vi "Enqeue message camera.vi"(8 "error in (no error)":errorcluster, 11 "RxTxCamera in":refnum<class "RxTxCamera.lvclass">) -> (0 "error out":errorcluster, 3 "RxTxCamera out":refnum<class "RxTxCamera.lvclass">)   [LabVIEW 2012, in "RxTxCamera.lvclass"]
uses:
  RxTxCamera.lvclass
  RxTx/RxTx.lvclass
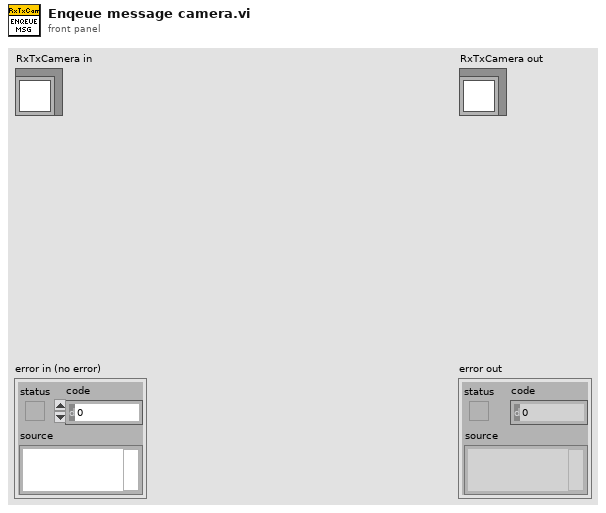
[diagram p1: front panel]
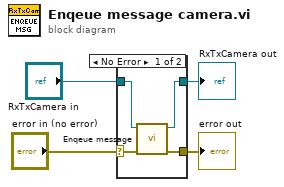
[diagram p0: block diagram]
diagram:
  n1 = case shown="No Error" "error in (no error)" {
    selector: "error in (no error)" -> [w6 w10]
    tunnel: [w5 w10] -> w3
    tunnel: [w7 w9] -> w1
    tunnel: "RxTxCamera in" -> [w8 w9]
    frame No Error {
      n2 = call "Enqeue message.vi"("error in (no error)"=w6, "RxTx in"=w8) -> ("error out"=w5:errorcluster, "RxTx out"=w7:refnum<class "RxTxCamera.lvclass">)  [unwired: 8 in]
    }
    frame Error {
    }
  }
  "error out" <- w3
  "RxTxCamera out" <- w1
